vi "ChangeFlag-Read.vi"(11 "ChangeFlagQ":refnum<queue>) -> (2 "Error Out":errorcluster, 3 "ChangeFlag":u64)   [LabVIEW 2017, in "Communicable State Machine.lvlib"]
uses:
  Communicable State Machine.lvlib
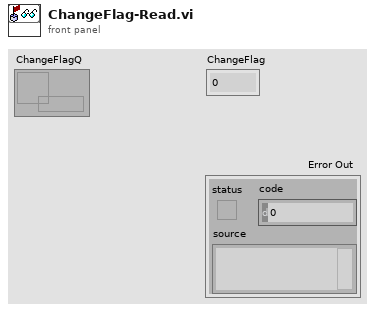
[diagram p1: front panel]
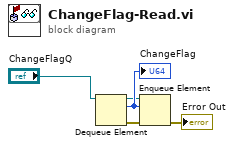
[diagram p0: block diagram]
diagram:
  n1 = Dequeue Element(queue="ChangeFlagQ") -> (queue out=w3:refnum<queue>, element=w4:u64, error out=w2:errorcluster)  [unwired: 2 in, 1 out]
  "ChangeFlag" <- w4
  n2 = Enqueue Element(queue=w3, element=w4, error in (no error)=w2) -> (error out=→"Error Out":errorcluster)  [unwired: 1 in, 2 out]
